vi "write memory.vi"(8 "error in (no error)":errorcluster, 10 "IQ data":u64[](array[numeric]), 11 "5785_3.2GHz_one channel in":refnum<class "5785_3.2GHz_one channel.lvclass">) -> (0 "error out":errorcluster, 3 "5785_3.2GHz_one channel out":refnum<class "5785_3.2GHz_one channel.lvclass">)   [LabVIEW 2021, in "5785_3.2GHz_one channel.lvclass"]
uses:
  5785_3.2GHz_one channel.lvclass
  5785_3.2GHz_one channel.lvclass/5785_3.2GHz_one channel.ctl
  <vilib>/rvi/interface/common/niFpgaWaitOnOcc.vi
  <vilib>/Utility/error.llb/Error Cluster From Error Code.vi
  <vilib>/rvi/errors/niLvFpgaAdjustHostInterfaceError.vi
  <vilib>/rvi/interface/nirviMethod/nirviMethod.xnode
  <vilib>/rvi/errors/niLvFpgaMergeErrorWithErrorCode.vi
  <vilib>/FPGAPlugInAG/Dynamic/niLvFpga_ConfigureFifo_Dynamic.vi
  <vilib>/FPGAPlugInAG/Dynamic/niLvFpga_WriteFifo_Dynamic.vi
  <vilib>/FPGAPlugInAG/Dynamic/niLvFpga_StopFifo_Dynamic.vi
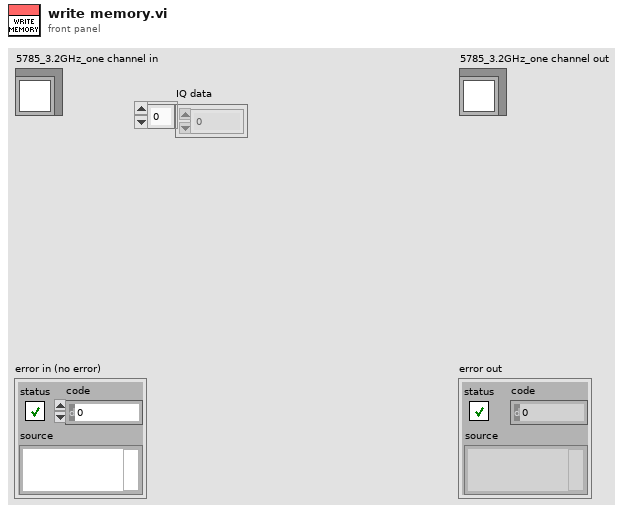
[diagram p1: front panel]
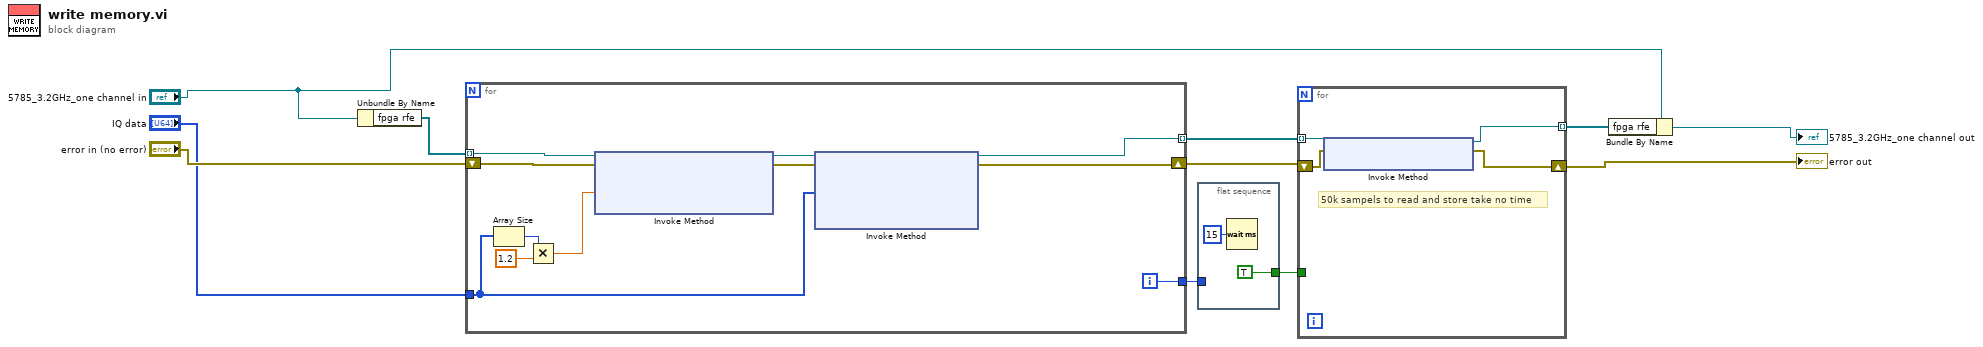
[diagram p0: block diagram]
diagram:
  n1 = Unbundle By Name("5785_3.2GHz_one channel in") -> ("fpga rfe"=w11:refnum<k20>[])
  n2 = for {
    tunnel: w11 -> [w16] mode=indexing
    tunnel: "IQ data" -> [w20]
    shift-right: [w21] -> w8
    shift-left: "error in (no error)" -> [w15]
    tunnel: [w22] -> w10 mode=indexing
    tunnel: [w12] -> w2
    i -> [w12]
    n3 = Array Size(array=w20) -> (size(s)=w19:i32)
    n4 = Multiply(x=w19, y=1.2) -> (x*y=w18:dbl)
    n5 = xnode "Invoke Method"("FPGA VI Reference In"=w16, "error in"=w15, "Requested Depth"=w18) -> ("FPGA VI Reference Out"=w14:refnum<k20>, "error out"=w13:errorcluster)  [unwired: 1 out]
    n6 = xnode "Invoke Method"("FPGA VI Reference In"=w14, "error in"=w13, "Data"=w20) -> ("FPGA VI Reference Out"=w22:refnum<k20>, "error out"=w21:errorcluster)  [unwired: 1 in, 1 out]
  }
  n7 = flat-sequence {
    tunnel: [TRUE] -> w7
    tunnel: w2 -> [_]
    frame #0 {
      n8 = Wait (ms)(milliseconds to wait=u32 15) -> ()  [unwired: 1 out]
    }
  }
  n9 = for {
    tunnel: w10 -> [w28] mode=indexing
    tunnel: [w26] -> w9 mode=indexing
    shift-right: [w25] -> w3
    shift-left: w8 -> [w27]
    tunnel: w7 -> [_]
    # "50k sampels to read and store take no time"
    n10 = xnode "Invoke Method"("FPGA VI Reference In"=w28, "error in"=w27) -> ("FPGA VI Reference Out"=w26:refnum<k20>, "error out"=w25:errorcluster)
  }
  "error out" <- w3
  n11 = Bundle By Name(cluster="5785_3.2GHz_one channel in", "fpga rfe"=w9) -> (→"5785_3.2GHz_one channel out":refnum<class "5785_3.2GHz_one channel.lvclass">)
